vi "open vi.vi"(7 "Show VI":bool=TRUE, 8 "error in":errorcluster, 9 "password":string, 10 "options":i32, 11 "VI Path":string) -> (0 "error out":errorcluster, 3 "vi id":string)   [LabVIEW 2020]
doc: "Open an existing LabVIEW VI and optional shows the block diagram to the user. Use the returned vi id with other tools to modify the VI. Use this Tool to get a reference to vi in order to modify the content."
uses:
  G-AI Core/G-AI Core.lvlib
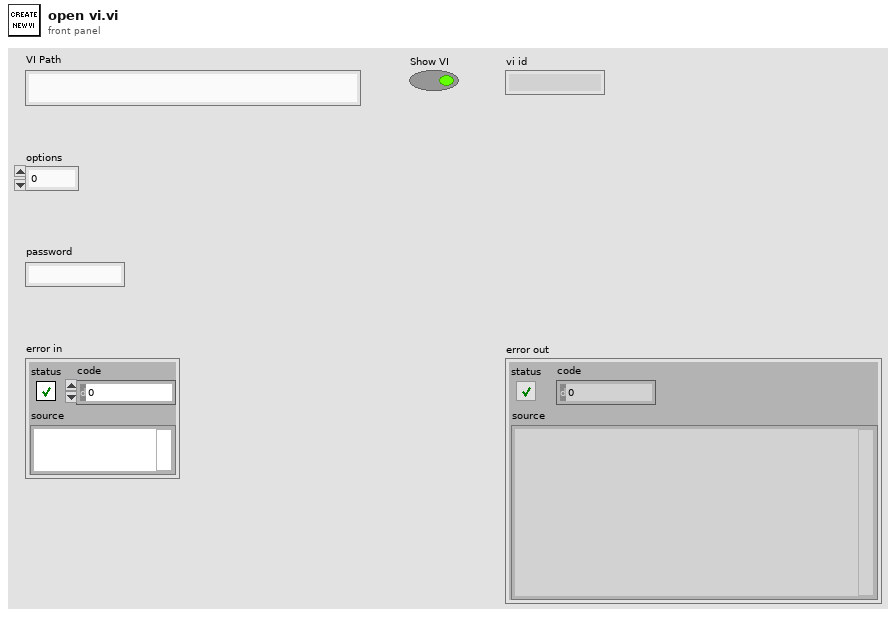
[diagram p1: front panel]
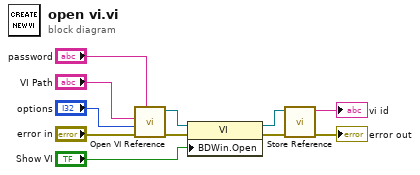
[diagram p0: block diagram]
diagram:
  n1 = call "Open VI Reference.vi"("password"="password", "error in"="error in", "options"="options", "VI Path"="VI Path") -> ("error out"=w11:errorcluster, "VI Refnum"=w10:refnum<vi>)  [unwired: 6 in]
  n2 = property class="VI"(reference=w10, error in=w11, "BDWin.Open"="Show VI") -> (reference out=w7:refnum<vi>, error out=w8:errorcluster)
  n3 = call "Store Reference.vi"("error in"=w8, "Reference"=w7) -> ("error out"=→"error out":errorcluster, "id"=→"vi id":string)  [unwired: 8 in]
